vi "DSF.Engine.Transceiver.Initialize.vi"(8 "error in (no error)":errorcluster, 10 "Transfer Groups":refnum<class "DSF.Engine.Transfer Group.lvclass">[](array[class]), 11 "UDP Transceiver in":refnum<class "DSF.Transceiver.UDP.lvclass">) -> (0 "error out":errorcluster, 3 "UDP Transceiver out":refnum<class "DSF.Transceiver.UDP.lvclass">)   [LabVIEW 2017, in "DSF.Transceiver.UDP.lvlib" / "DSF.Transceiver.UDP.lvclass"]
uses:
  DSF.Transceiver.UDP.lvclass
  Built/DSF.Engine.lvlibp/Engine/Classes/Transfer/DSF.Engine.Transfer Group.lvclass
  DSF.Transceiver.UDP.lvclass/DSF.Transceiver.UDP.ctl
  DSF.Transceiver.UDP.Tx Parameters.ctl
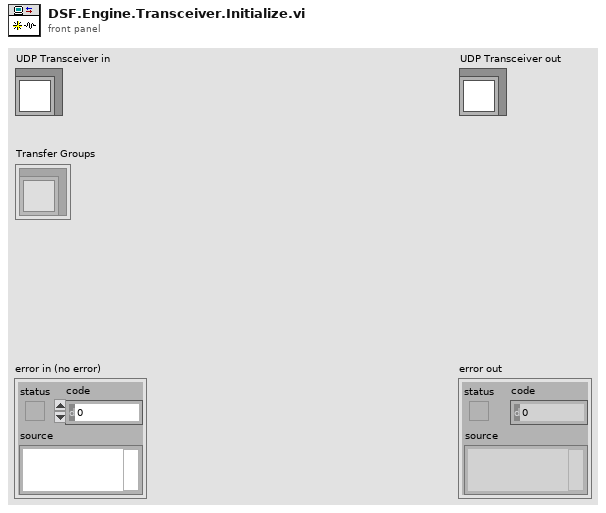
[diagram p1: front panel]
types:
  T1 = cluster{"destination ip address":string, "destination port":u16, "source port":u16}[]
  T2 = typedef "DSF.Transceiver.UDP.lvlib/DSF.Transceiver.UDP.lvclass/DSF.Transceiver.UDP.Tx Parameters.ctl" = cluster{"connection ID":refnum<k16>, "address":u32, "port or service name":u16}
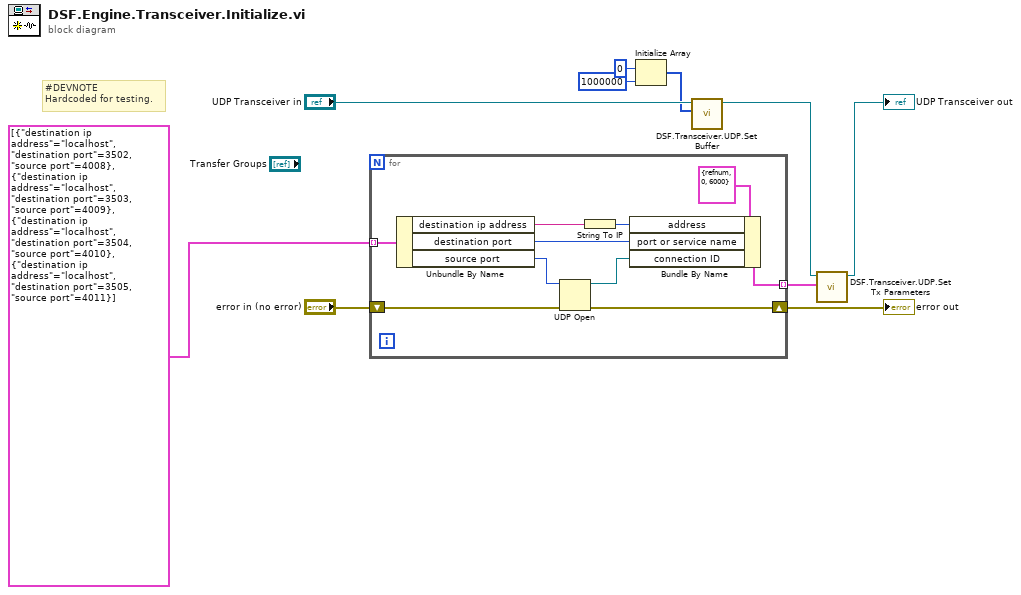
[diagram p0: block diagram]
diagram:
  # "#DEVNOTE\nHardcoded for testing."
  n1 = for {
    shift-right: [w19] -> w8
    shift-left: "error in (no error)" -> [w20]
    tunnel: [w16] -> w7 mode=indexing
    tunnel: T1 [{"destination ip address"="localhost", "destination port"=3502, "source port"=4008}, {"destination ip address"="localhost", "destination port"=3503, "source port"=4009}, {"destination ip address"="localhost", "destination port"=3504, "source port"=4010}, {"destination ip address"="localhost", "destination port"=3505, "source port"=4011}] -> [w14] mode=indexing
    n2 = Unbundle By Name(w14) -> ("destination ip address"=w11:string, "destination port"=w12:u16, "source port"=w13:u16)
    n3 = UDP Open(8:w20, 11:w13) -> (port=w17:refnum<k16>, 0:w19:errorcluster)  [unwired: 3 in, 1 out]
    n4 = String To IP(1:w11) -> (0:w15:u32)
    n5 = Bundle By Name(cluster=T2 {"connection ID"=refnum, "address"=0, "port or service name"=6000} ("Tx"), "address"=w15, "port or service name"=w12, "connection ID"=w17) -> (w16:T2)
  }
  "error out" <- w8
  n6 = Initialize Array(u8 0 ("element"), 1000000 ("dimension size")) -> (w3:u8[])
  n7 = call "DSF.Transceiver.UDP.Set Buffer.vi"("buffer"=w3, "DSF.Transceiver.UDP in"="UDP Transceiver in") -> ("DSF.Transceiver.UDP out"=w4:refnum<class "DSF.Transceiver.UDP.lvclass">)  [unwired: 9 in]
  n8 = call "DSF.Transceiver.UDP.Set Tx Parameters.vi"("Tx parameters"=w7, "DSF.Transceiver.UDP in"=w4) -> ("DSF.Transceiver.UDP out"=→"UDP Transceiver out":refnum<class "DSF.Transceiver.UDP.lvclass">)  [unwired: 9 in]
